vi "Pin Position Facade.vi"(0 "Data In":T6, 2 "Display State In":T3, 3 "Container State":T5) -> (6 "Data Out":T6, 7 "Display State Out":T3, 8 "Action":T2)   [LabVIEW 2013, in "Pin Position.xctl"]
uses:
  Pin Position.xctl
  Popups/Selected Pin Positions.ctl
  Pin Position Data.ctl
  lib/Data Access Objects/Metadata/Pin Positions.ctl
  <vilib>/_xctls/Container State.ctl
  Pin Position State.ctl
  lib/Data Access Objects/Application/Number Of LBCBs.ctl
  <vilib>/_xctls/Action.ctl
  lib/Data Access Objects/Metadata/Persistant DAO Actions.ctl
  lib/Data Access Objects/Metadata/LBCB Number.ctl
  <vilib>/_xctls/XControlSupport.lvlib
panel:
  in  "LBCB Position Tab":enum32{"LBCB 1", "LBCB 2"}(tab)
  in  "LBCB Position L1":T1
  in  "LBCB Position L2":T1
  # "Fixed"
  # "Platten"
  # "X"
  # "Z"
  # "X"
  # "Z"
  # "Y"
  # "Y"
  # "Fixed"
  # "Platten"
  # "X"
  # "Z"
  # "X"
  # "Z"
  # "Y"
  # "Y"
  # "Fixed"
  # "Platten"
  # "X"
  # "Z"
  # "X"
  # "Z"
  # "Y"
  # "Y"
  # "Fixed"
  # "Platten"
  # "X"
  # "Z"
  # "X"
  # "Z"
  # "Y"
  # "Y"
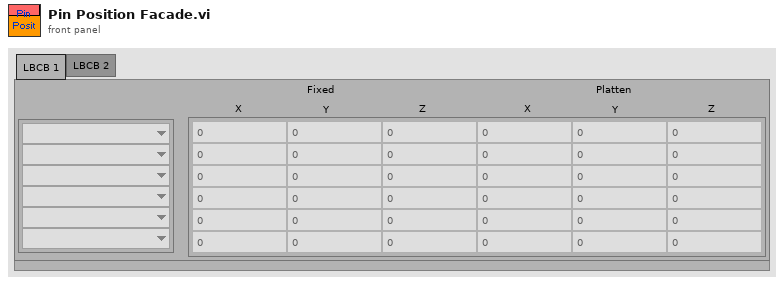
[diagram p1: front panel]
types:
  T1 = typedef "Selected Pin Positions.ctl" = cluster{"Pin Positions":dbl[][], "Row Labels":u16[]}
  T2 = typedef "XControlSupport.lvlib/Action.ctl" = cluster{"Data Changed?":bool, "State Changed?":bool, "Action Name":string}
  T3 = typedef "Pin Position.xctl/Pin Position State.ctl" = cluster{"Number  of LBCBs":T4, "RowNames":string[]}
  T4 = typedef "Number Of LBCBs.ctl" = enum16{"1", "2"}
  T5 = typedef "XControlSupport.lvlib/Container State.ctl" = cluster{"Indicator?":bool, "Run Mode?":bool, " Refnum":refnum<vi>}
  T6 = typedef "Pin Position.xctl/Pin Position Data.ctl" = T7[]
  T7 = typedef "Pin Positions.ctl" = cluster{"Pin Positions":dbl[][], "Row Labels":string[]}
  T8 = enum8{"Enabled", "Disabled", "Disabled and Grayed Out"}
  T9 = typedef "LBCB Number.ctl" = enum16{"LBCB1", "LBCB2"}
  T10 = typedef "Persistant DAO Actions.ctl" = enum16{"Init", "Get", "Set", "Load", "Save"}
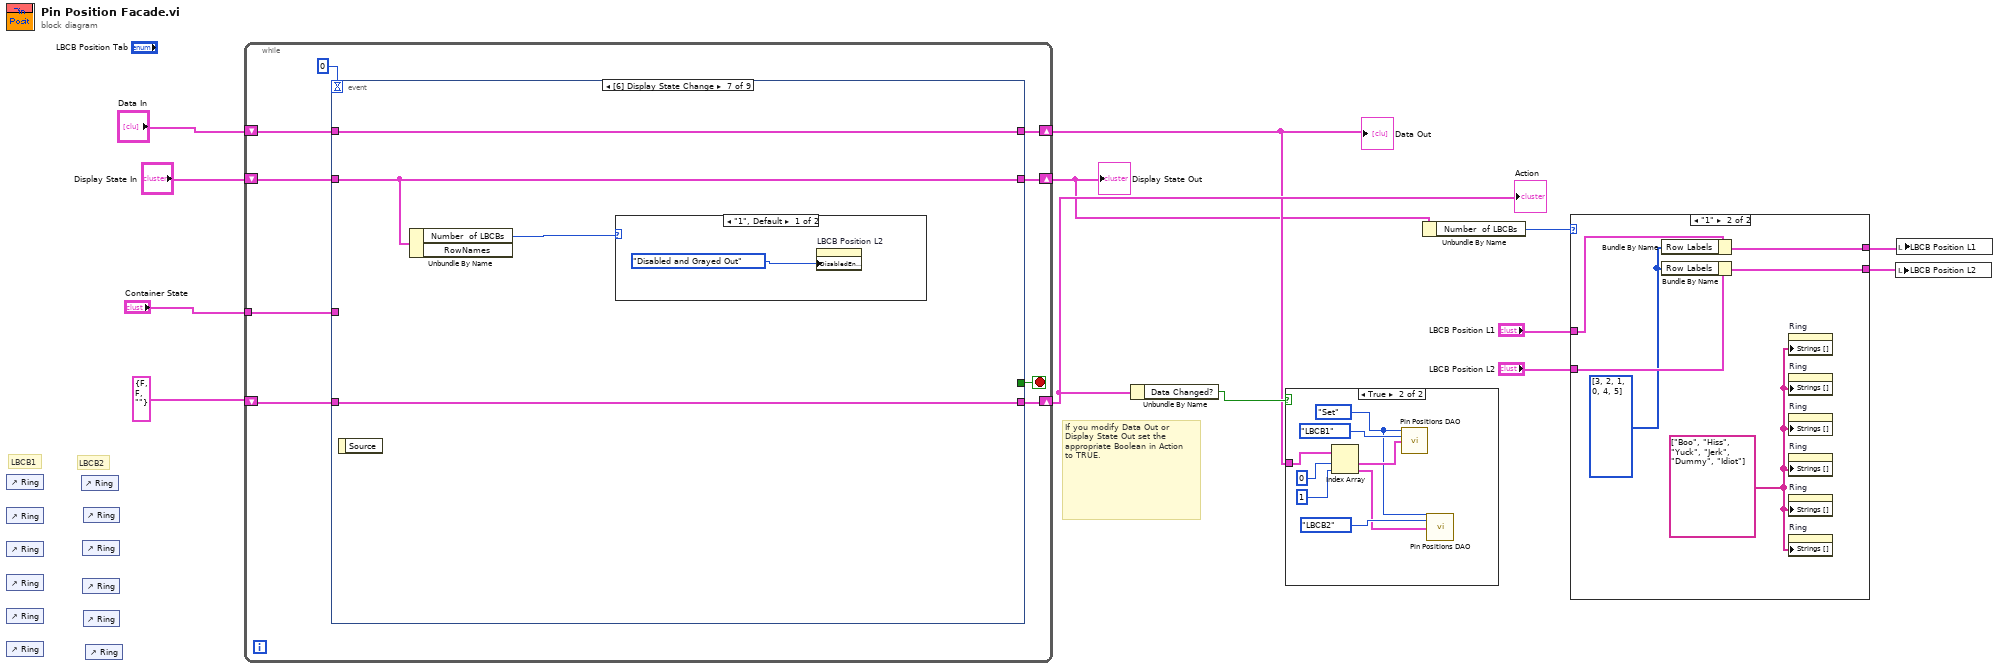
[diagram p0: block diagram]
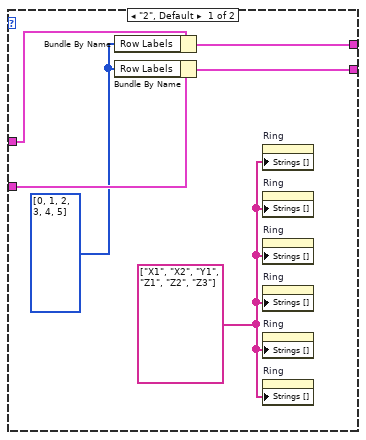
[diagram p2: hidden frame]
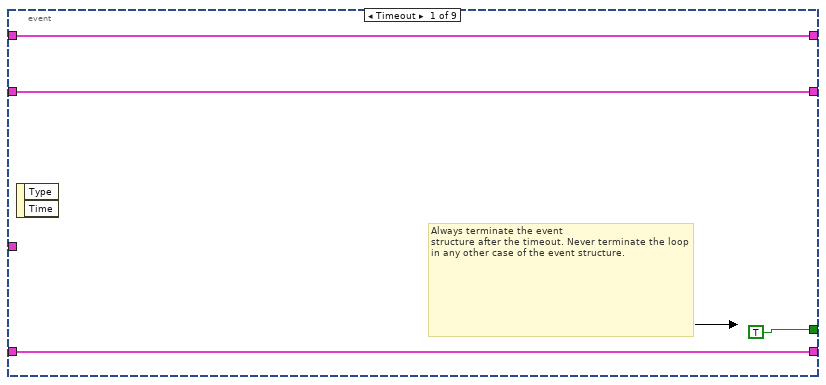
[diagram p4: hidden frame]
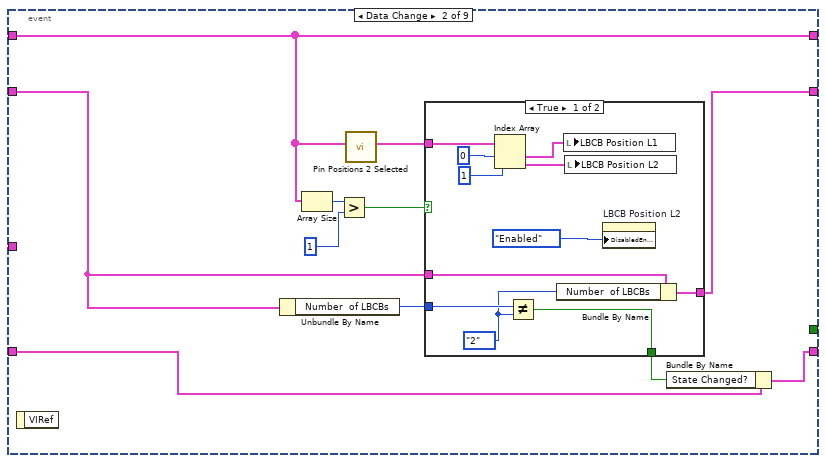
[diagram p5: hidden frame]
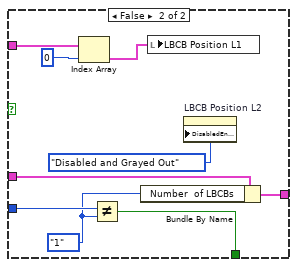
[diagram p6: hidden frame]
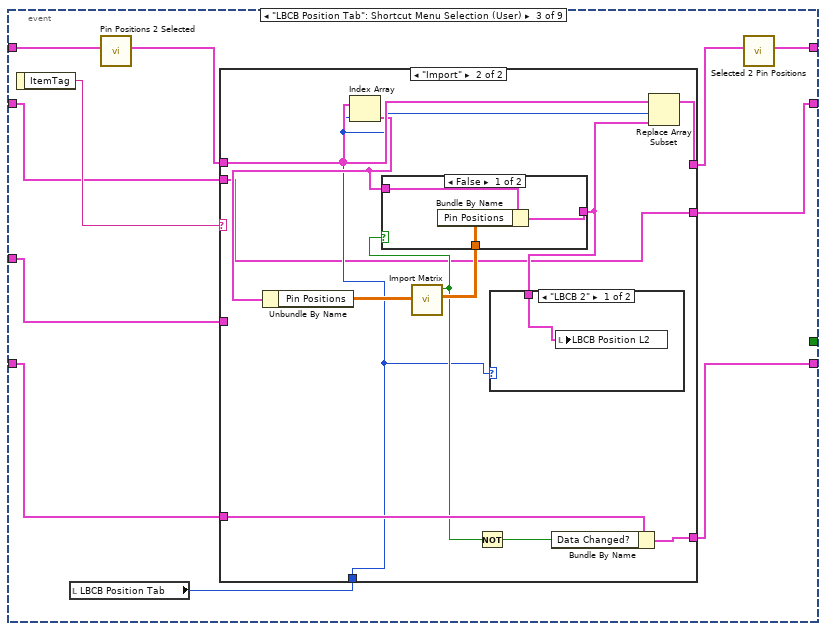
[diagram p7: hidden frame]
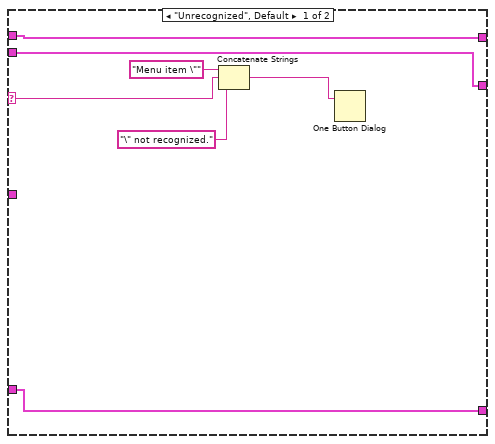
[diagram p8: hidden frame]
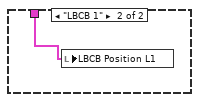
[diagram p9: hidden frame]
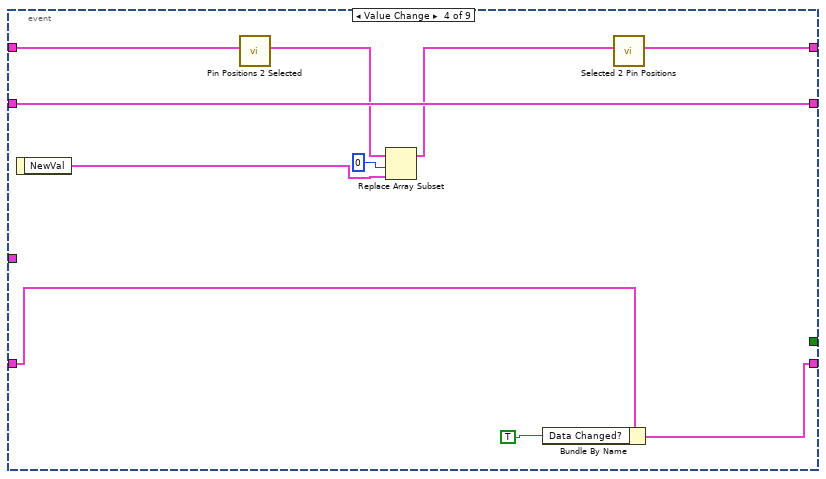
[diagram p11: hidden frame]
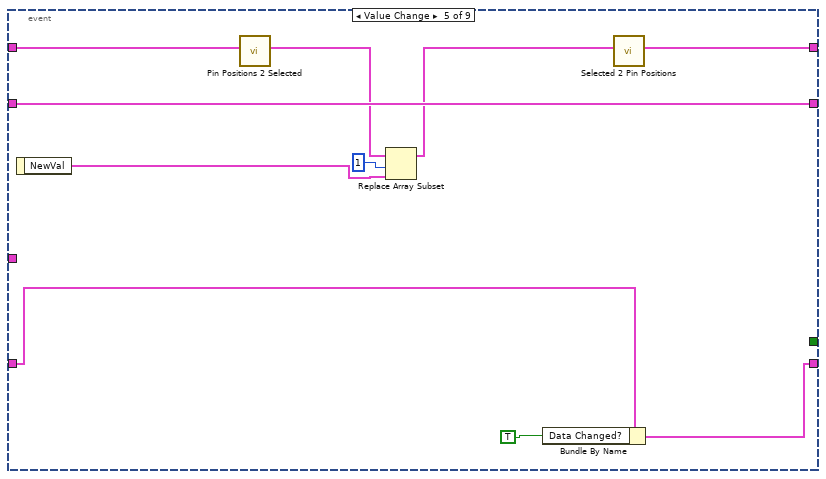
[diagram p12: hidden frame]
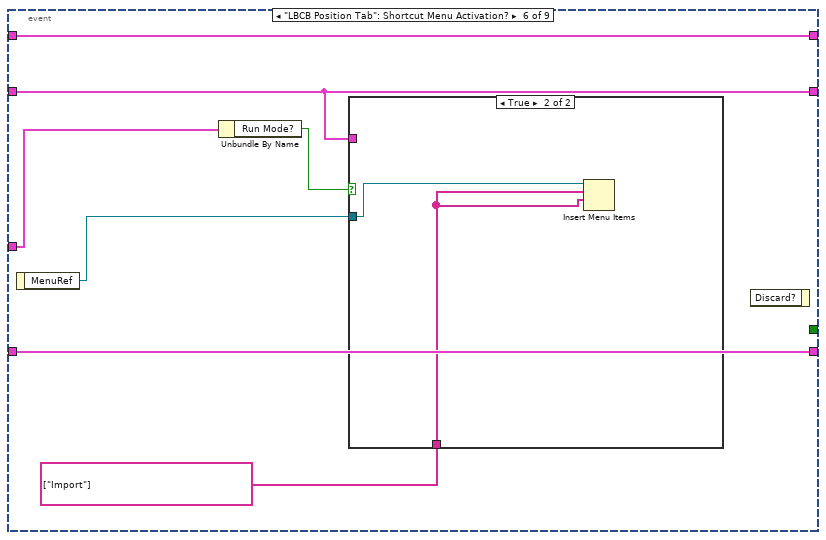
[diagram p13: hidden frame]
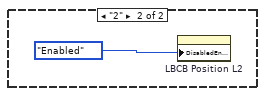
[diagram p15: hidden frame]
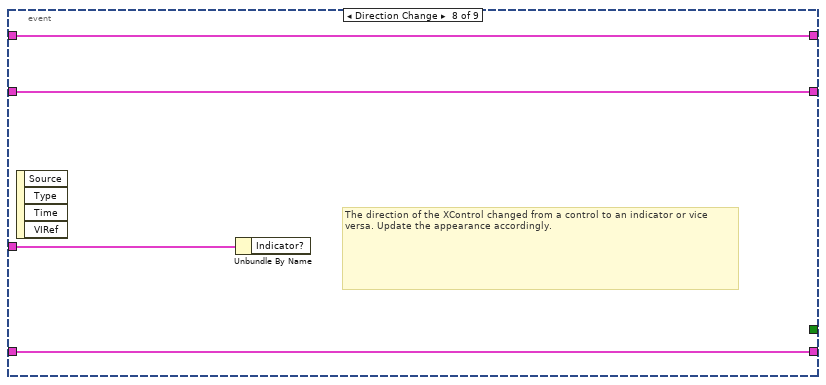
[diagram p16: hidden frame]
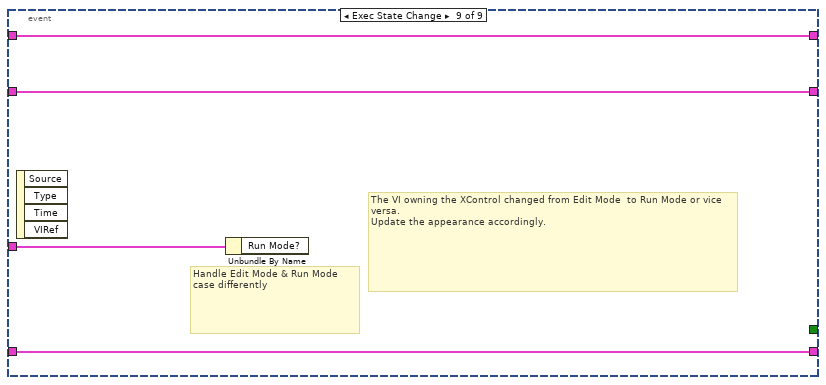
[diagram p17: hidden frame]
diagram:
  # "LBCB2"
  # "LBCB1"
  # "If you modify Data Out or\nDisplay State Out set the\nappropriate Boolean in Action\nto TRUE."
  n1 = control-ref of="Ring"() -> ()  [unwired: 1 out]
  n2 = control-ref of="Ring"() -> ()  [unwired: 1 out]
  n3 = control-ref of="Ring"() -> ()  [unwired: 1 out]
  n4 = control-ref of="Ring"() -> ()  [unwired: 1 out]
  n5 = control-ref of="Ring"() -> ()  [unwired: 1 out]
  n6 = control-ref of="Ring"() -> ()  [unwired: 1 out]
  n7 = control-ref of="Ring"() -> ()  [unwired: 1 out]
  n8 = control-ref of="Ring"() -> ()  [unwired: 1 out]
  n9 = control-ref of="Ring"() -> ()  [unwired: 1 out]
  n10 = control-ref of="Ring"() -> ()  [unwired: 1 out]
  n11 = control-ref of="Ring"() -> ()  [unwired: 1 out]
  n12 = control-ref of="Ring"() -> ()  [unwired: 1 out]
  n13 = while {
    shift-right: [w21] -> w2
    shift-left: "Display State In" -> [w22]
    tunnel: "Container State" -> [w18]
    shift-right: [w16] -> w8
    shift-left: "Data In" -> [w17]
    shift-right: [w14] -> w9
    shift-left: T2 {"Data Changed?"=FALSE, "State Changed?"=FALSE, "Action Name"=""} ("Action") -> [w15]
    stop <- w20 stop-if-true
    n14 = event shown="[6] Display State Change" {
      selector: _ -> [_ _ _ _ _ _ _ _ _]
      dyn-events: _ -> [_ _ _ _ _ _ _ _ _]
      timeout: 0 -> [_ _ _ _ _ _ _ _ _]
      tunnel: w22 -> [w24 w29 w59 w103 w113 w114 w123 w131 w135]
      tunnel: [w24 w28 w58 w103 w113 w114 w123 w131 w135] -> w21
      tunnel: [TRUE _ _ _ _ _ _ _ _] -> w20
      tunnel: w18 -> [_ _ w60 _ _ w117 _ w132 w136]
      tunnel: w17 -> [w23 w32 w66 w99 w109 w115 w126 w130 w134]
      tunnel: [w23 w32 w62 w96 w106 w115 w126 w130 w134] -> w16
      tunnel: [w25 w30 w64 w94 w104 w120 w125 w129 w133] -> w14
      tunnel: w15 -> [w25 w31 w68 w95 w105 w120 w125 w129 w133]
      event Timeout {
        # "Always terminate the event\nstructure after the timeout. Never terminate the loop in any other case of the event structure."
        n15 = event-data() -> ()  [unwired: 1 in, 2 out]
      }
      event Data Change {
        n16 = event-data() -> ()  [unwired: 1 in, 1 out]
        n17 = Unbundle By Name(w29) -> ("Number  of LBCBs"=w36:T4)
        n18 = Array Size(array=w32) -> (size(s)=w33:i32)
        n19 = Greater?(x=w33, y=1) -> (0:w35:bool)
        n20 = call "Pin Positions 2 Selected.vi"("Pin"=w32) -> ("Selected"=w27:T1[])  [unwired: 10 in]
        n21 = case shown="True" w35 {
          tunnel: w27 -> [w48 w57]
          tunnel: w29 -> [w42 w53]
          tunnel: w36 -> [w43 w54]
          tunnel: [w40 w51] -> w37
          tunnel: [w39 w50] -> w28
          frame True {
            w41 = Number_Of_LBCBs."2" ("y")
            n22 = Index Array(array=w48, index #1=0 ("index"), index #2=1 ("index")) -> (element #1=w45:T1, element #2=w44:T1)
            n23 = Not Equal?(x=w43, y=w41) -> (x != y?=w40:bool)
            n24 = Bundle By Name(cluster=w42, "Number  of LBCBs"=w41) -> (w39:T3)
            n25 = local write "LBCB Position L1"(w45) -> ()
            n26 = local write "LBCB Position L2"(w44) -> ()
            n27 = property on="LBCB Position L2" class="Clust (strict)"("DisabledEnum"=T8."Enabled" ("Disabled")) -> ()  [unwired: 2 in, 2 out]
          }
          frame False {
            w52 = Number_Of_LBCBs."1" ("y")
            n28 = Index Array(array=w57, index=0) -> (element=w55:T1)
            n29 = Not Equal?(x=w54, y=w52) -> (x != y?=w51:bool)
            n30 = Bundle By Name(cluster=w53, "Number  of LBCBs"=w52) -> (w50:T3)
            n31 = local write "LBCB Position L1"(w55) -> ()
            n32 = property on="LBCB Position L2" class="Clust (strict)"("DisabledEnum"=T8."Disabled and Grayed Out" ("Disabled")) -> ()  [unwired: 2 in, 2 out]
          }
        }
        n33 = Bundle By Name(cluster=w31, "State Changed?"=w37) -> (w30:T2)
      }
      event "LBCB Position Tab": Shortcut Menu Selection (User) {
        n34 = event-data() -> ("ItemTag"=w67:string)  [unwired: 1 in]
        n35 = local read "LBCB Position Tab"() -> (w61:enum32{"LBCB 1", "LBCB 2"})
        n36 = call "Pin Positions 2 Selected.vi"("Pin"=w66) -> ("Selected"=w63:T1[])  [unwired: 10 in]
        n37 = case shown="\"Import\"" w67 {
          selector: w67 -> [w73 _]
          tunnel: w63 -> [w71 w87]
          tunnel: [w71 w86] -> w65
          tunnel: w68 -> [w70 w82]
          tunnel: [w70 w81] -> w64
          tunnel: w61 -> [_ w77]
          tunnel: w60 -> [_ _]
          tunnel: w59 -> [w69 w76]
          tunnel: [w69 w76] -> w58
          frame "Unrecognized", Default {
            n38 = Concatenate Strings("Menu item \"" ("string"), w73, "\" not recognized." ("string")) -> (w72:string)
            n39 = One Button Dialog(message=w72) -> ()  [unwired: 1 in, 1 out]
          }
          frame "Import" {
            n40 = Index Array(array=w87, index=w77) -> (element=w85:T1)
            n41 = Unbundle By Name(w85) -> ("Pin Positions"=w84:dbl[][])
            n42 = call "Import Matrix.vi"("PinPositions In"=w84) -> ("PinPositions Out"=w83:dbl[][], "Canceled"=w80:bool)  [unwired: 9 in]
            n43 = case shown="False" w80 {
              tunnel: [w92 w93] -> w78
              tunnel: w85 -> [w91 w93]
              tunnel: w83 -> [w90 _]
              frame False {
                n44 = Bundle By Name(cluster=w91, "Pin Positions"=w90) -> (w92:T1)
              }
              frame True {
              }
            }
            n45 = Not(x=w80) -> (.not. x?=w79:bool)
            n46 = case shown="\"LBCB 2\"" w77 {
              tunnel: w78 -> [w88 w89]
              frame "LBCB 2" {
                n47 = local write "LBCB Position L2"(w88) -> ()
              }
              frame "LBCB 1" {
                n48 = local write "LBCB Position L1"(w89) -> ()
              }
            }
            n49 = Bundle By Name(cluster=w82, "Data Changed?"=w79) -> (w81:T2)
            n50 = Replace Array Subset(array=w87, new element=w78, index=w77) -> (w86:T1[])
          }
        }
        n51 = call "Selected 2 Pin Positions.vi"("Selected"=w65) -> ("Pin"=w62:T7[])  [unwired: 10 in]
      }
      event Value Change {
        n52 = event-data() -> ("NewVal"=w100:T1)  [unwired: 1 in]
        n53 = call "Pin Positions 2 Selected.vi"("Pin"=w99) -> ("Selected"=w98:T1[])  [unwired: 10 in]
        n54 = Replace Array Subset(array=w98, new element=w100, index=0) -> (w97:T1[])
        n55 = Bundle By Name(cluster=w95, "Data Changed?"=TRUE) -> (w94:T2)
        n56 = call "Selected 2 Pin Positions.vi"("Selected"=w97) -> ("Pin"=w96:T7[])  [unwired: 10 in]
      }
      event Value Change {
        n57 = event-data() -> ("NewVal"=w110:T1)  [unwired: 1 in]
        n58 = call "Pin Positions 2 Selected.vi"("Pin"=w109) -> ("Selected"=w108:T1[])  [unwired: 10 in]
        n59 = Replace Array Subset(array=w108, new element=w110, index=1) -> (w107:T1[])
        n60 = Bundle By Name(cluster=w105, "Data Changed?"=TRUE) -> (w104:T2)
        n61 = call "Selected 2 Pin Positions.vi"("Selected"=w107) -> ("Pin"=w106:T7[])  [unwired: 10 in]
      }
      event "LBCB Position Tab": Shortcut Menu Activation? {
        n62 = event-data() -> ("MenuRef"=w116:refnum<k9>)  [unwired: 1 in]
        n63 = Unbundle By Name(w117) -> ("Run Mode?"=w118:bool)
        n64 = case shown="True" w118 {
          tunnel: w116 -> [_ w122]
          tunnel: string[] ["Import"] -> [_ w121]
          tunnel: w114 -> [_ _]
          frame False {
          }
          frame True {
            n65 = Insert Menu Items(7:w121, 8:w121, 9:w122) -> ()  [unwired: 3 in, 3 out]
          }
        }
        n66 = event-data() -> ()  [unwired: 2 in, 1 out]
      }
      event Display State Change {
        n67 = event-data() -> ()  [unwired: 1 in, 1 out]
        n68 = Unbundle By Name(w123) -> ("Number  of LBCBs"=w124:T4)  [unwired: 1 out]
        n69 = case shown="\"1\", Default" w124 {
          frame "1", Default {
            n70 = property on="LBCB Position L2" class="Clust (strict)"("DisabledEnum"=T8."Disabled and Grayed Out" ("Disabled")) -> ()  [unwired: 2 in, 2 out]
          }
          frame "2" {
            n71 = property on="LBCB Position L2" class="Clust (strict)"("DisabledEnum"=T8."Enabled" ("Disabled")) -> ()  [unwired: 2 in, 2 out]
          }
        }
      }
      event Direction Change {
        # "The direction of the XControl changed from a control to an indicator or vice versa. Update the appearance accordingly."
        n72 = event-data() -> ()  [unwired: 1 in, 4 out]
        n73 = Unbundle By Name(w132) -> ()  [unwired: 1 out]
      }
      event Exec State Change {
        # "The VI owning the XControl changed from Edit Mode  to Run Mode or vice versa.\nUpdate the appearance accordingly."
        # "Handle Edit Mode & Run Mode\ncase differently"
        n74 = event-data() -> ()  [unwired: 1 in, 4 out]
        n75 = Unbundle By Name(w136) -> ()  [unwired: 1 out]
      }
    }
  }
  "Display State Out" <- w2
  "Data Out" <- w8
  "Action" <- w9
  n76 = Unbundle By Name(w9) -> ("Data Changed?"=w10:bool)
  n77 = case shown="True" w10 {
    tunnel: w8 -> [_ w141]
    frame False {
    }
    frame True {
      w139 = Persistant_DAO_Actions."Set" ("LBCB Settings Actions")
      n78 = Index Array(array=w141, index #1=0 ("index"), index #2=1 ("index")) -> (element #1=w140:T7, element #2=w137:T7)
      n79 = call "Pin Positions DAO.vi"("LBCB Settings Actions"=w139, "LBCB Number"=LBCB_Number."LBCB1", "LBCB Pins In"=w140) -> ()  [unwired: 10 in, 3 out]
      n80 = call "Pin Positions DAO.vi"("LBCB Settings Actions"=w139, "LBCB Number"=LBCB_Number."LBCB2", "LBCB Pins In"=w137) -> ()  [unwired: 10 in, 3 out]
    }
  }
  n81 = Unbundle By Name(w2) -> ("Number  of LBCBs"=w7:T4)
  n82 = case shown="\"1\"" w7 {
    tunnel: "LBCB Position L1" -> [w149 w155]
    tunnel: "LBCB Position L2" -> [w146 w152]
    tunnel: [w148 w154] -> w4
    tunnel: [w147 w153] -> w3
    frame "2", Default {
      w145 = i32[] [0, 1, 2, 3, 4, 5]
      w150 = string[] ["X1", "X2", "Y1", "Z1", "Z2", "Z3"]
      n83 = Bundle By Name(cluster=w149, "Row Labels"=w145) -> (w148:T1)
      n84 = Bundle By Name(cluster=w146, "Row Labels"=w145) -> (w147:T1)
      n85 = property on="Ring" class="Ring (strict)"("Strings []"=w150) -> ()  [unwired: 2 in, 2 out]
      n86 = property on="Ring" class="Ring (strict)"("Strings []"=w150) -> ()  [unwired: 2 in, 2 out]
      n87 = property on="Ring" class="Ring (strict)"("Strings []"=w150) -> ()  [unwired: 2 in, 2 out]
      n88 = property on="Ring" class="Ring (strict)"("Strings []"=w150) -> ()  [unwired: 2 in, 2 out]
      n89 = property on="Ring" class="Ring (strict)"("Strings []"=w150) -> ()  [unwired: 2 in, 2 out]
      n90 = property on="Ring" class="Ring (strict)"("Strings []"=w150) -> ()  [unwired: 2 in, 2 out]
    }
    frame "1" {
      w151 = i32[] [3, 2, 1, 0, 4, 5]
      w156 = string[] ["Boo", "Hiss", "Yuck", "Jerk", "Dummy", "Idiot"]
      n91 = Bundle By Name(cluster=w155, "Row Labels"=w151) -> (w154:T1)
      n92 = Bundle By Name(cluster=w152, "Row Labels"=w151) -> (w153:T1)
      n93 = property on="Ring" class="Ring (strict)"("Strings []"=w156) -> ()  [unwired: 2 in, 2 out]
      n94 = property on="Ring" class="Ring (strict)"("Strings []"=w156) -> ()  [unwired: 2 in, 2 out]
      n95 = property on="Ring" class="Ring (strict)"("Strings []"=w156) -> ()  [unwired: 2 in, 2 out]
      n96 = property on="Ring" class="Ring (strict)"("Strings []"=w156) -> ()  [unwired: 2 in, 2 out]
      n97 = property on="Ring" class="Ring (strict)"("Strings []"=w156) -> ()  [unwired: 2 in, 2 out]
      n98 = property on="Ring" class="Ring (strict)"("Strings []"=w156) -> ()  [unwired: 2 in, 2 out]
    }
  }
  n99 = local write "LBCB Position L2"(w3) -> ()
  n100 = local write "LBCB Position L1"(w4) -> ()
